vi "myRIOXC Set Cursor.vi"(9 "Cursor":u16, 10 "Container State":T1, 11 "PIN Ref":refnum<vi>) -> ()   [LabVIEW 2021]
uses:
  <vilib>/_xctls/Container State.ctl
  <vilib>/Utility/cursorutil.llb/Set Cursor (Icon Pict).vi
  <vilib>/_xctls/XControlSupport.lvlib
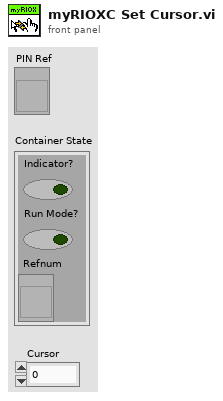
[diagram p1: front panel]
types:
  T1 = typedef "XControlSupport.lvlib/Container State.ctl" = cluster{"Indicator?":bool, "Run Mode?":bool, " Refnum":refnum<vi>}
  T2 = enum8{"Enabled", "Disabled", "Disabled and Grayed Out"}
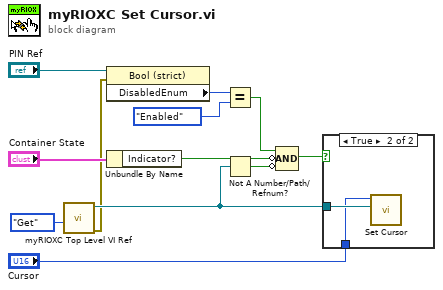
[diagram p0: block diagram]
diagram:
  n1 = call <vilib>:"myRIOXC Top Level VI Ref.vi"("Action"=enum16{"Get", "Set"}."Get") -> ("error out"=w1:errorcluster, "Top Level VI Ref out"=w10:refnum<vi>)  [unwired: 9 in]
  n2 = property class="Bool (strict)"(reference="PIN Ref", error in=w1) -> ("DisabledEnum"=w3:T2)  [unwired: 2 out]
  n3 = Unbundle By Name("Container State") -> ("Indicator?"=w11:bool)
  n4 = Equal?(x=w3, y=T2."Enabled" ("Disabled")) -> (x = y?=w7:bool)
  n5 = Not A Number/Path/Refnum?(number/path/refnum=w10) -> (NaN/Path/Refnum?=w12:bool)
  n6 = Compound Arithmetic op=AND(w7, invert w11, invert w12) -> (w8:bool)
  n7 = case shown="True" w8 {
    tunnel: w10 -> [_ w14]
    tunnel: "Cursor" -> [_ w13]
    frame False {
    }
    frame True {
      n8 = call-poly <vilib>:"Set Cursor.vi"("VI reference (current VI)"=w14, "icon"=w13) -> ()  [unwired: 8 in, 2 out]
    }
  }
